vi "Prepare Loggers.vi"(6 "Groups":string[](array[string]), 8 "error in (no error)":errorcluster, 9 "Series":string, 10 "Folder":path, 11 "Log Manager Module in":refnum<class "Log Manager Module.lvclass">) -> (0 "error out":errorcluster, 3 "Log Manager Module out":refnum<class "Log Manager Module.lvclass">)   [LabVIEW 2020, in "VolatusData.lvlib" / "Log Manager Module.lvclass"]
uses:
  Log Manager Module.lvclass
  C:/dev/lv20CE/relink/lv-volatus/Volatus/Module/Module.lvclass
  Prepare Log.ctl
  Log Manager Module.lvclass/Log Manager Module.ctl
  Volatus/Event Level.ctl
  Volatus/Module/Module.lvclass/Module.ctl
  Logger State.ctl
  Volatus/Module/Module.lvclass
  VolatusData.lvlib
  Volatus/Volatus.lvlib
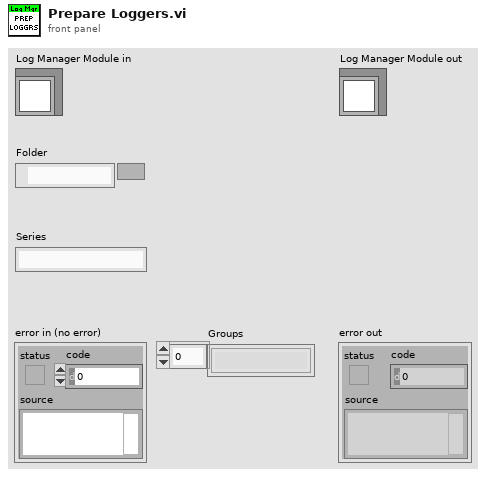
[diagram p1: front panel]
types:
  T1 = typedef "VolatusData.lvlib/Prepare Log.ctl" = cluster{"Folder":path, "Series":string}
  T2 = typedef "VolatusData.lvlib/Log Manager Module.lvclass/Group Info.ctl" = cluster{"Name":string, "Loggers":map{string, T3}}
  T3 = typedef "VolatusData.lvlib/Log Manager Module.lvclass/Logger.ctl" = cluster{"ID":string, "MsgQ":refnum<class "MessageQ.lvclass">, "State":T4, "Group":string}
  T4 = typedef "VolatusData.lvlib/Logger State.ctl" = enum16{"Unknown", "Idle", "Preparing", "Ready", "Logging", "Stopping"}
  T5 = typedef "Volatus.lvlib/Event Level.ctl" = enum16{"Debug", "Info", "Warning", "Error"}
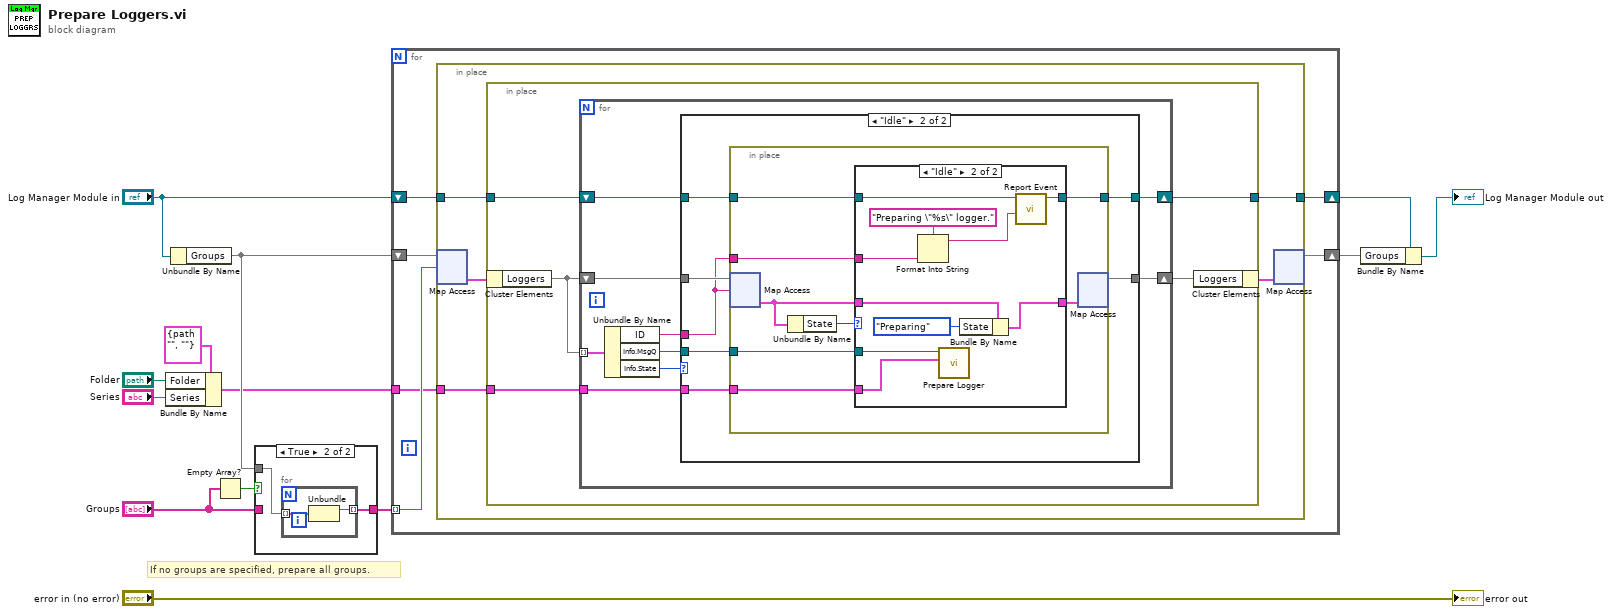
[diagram p0: block diagram]
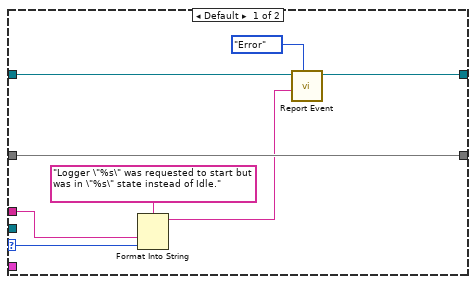
[diagram p2: hidden frame]
diagram:
  # "If no groups are specified, prepare all groups."
  n1 = Bundle By Name(cluster=T1 {"Folder"=path "", "Series"=""} ("Prepare Log"), "Folder"="Folder", "Series"="Series") -> (w1:T1)
  n2 = Unbundle By Name("Log Manager Module in") -> ("Groups"=w4:map{string, T2})
  n3 = Empty Array?(array="Groups") -> (empty?=w6:bool)
  n4 = case shown="True" w6 {
    tunnel: "Groups" -> [w14 _]
    tunnel: w4 -> [_ w16]
    tunnel: [w14 w15] -> w3
    frame False {
    }
    frame True {
      n5 = for {
        tunnel: w16 -> [w18] mode=indexing
        tunnel: [w17] -> w15 mode=indexing
        n6 = Unbundle(w18) -> ("Name"=w17:string)  [unwired: 1 out]
      }
    }
  }
  n7 = for {
    shift-right: [w23] -> w7
    shift-left: "Log Manager Module in" -> [w24]
    shift-right: [w20] -> w2
    shift-left: w4 -> [w22]
    tunnel: w3 -> [w21] mode=indexing
    tunnel: w1 -> [w19]
    n8 = in-place {
      in-place-border: w24 -> [w29]
      in-place-border: [w28] -> w23
      in-place-border: w19 -> [w25]
      n9 = in-place-map #1(w22, w21) -> (w27:T2)  [unwired: 1 in, 1 out]
      n10 = in-place {
        in-place-border: w29 -> [w34]
        in-place-border: [w33] -> w28
        in-place-border: w25 -> [w30]
        n11 = in-place-cluster #2(w27) -> ("Loggers"=w32:map{string, T3})
        n12 = for {
          tunnel: w32 -> [w43] mode=indexing
          shift-right: [w41] -> w31
          shift-left: w32 -> [w42]
          shift-right: [w38] -> w33
          shift-left: w34 -> [w39]
          tunnel: w30 -> [w35]
          n13 = Unbundle By Name(w43) -> ("ID"=w37:string, "Info.MsgQ"=w40:refnum<class "MessageQ.lvclass">, "Info.State"=w36:T4)
          n14 = case shown="\"Idle\"" w36 {
            selector: w36 -> [w46 _]
            tunnel: w42 -> [w49 w58]
            tunnel: [w49 w57] -> w41
            tunnel: w40 -> [_ w56]
            tunnel: w39 -> [w51 w55]
            tunnel: [w50 w54] -> w38
            tunnel: w37 -> [w45 w53]
            tunnel: w35 -> [_ w52]
            frame Default {
              n15 = Format Into String(format string="Logger \"%s\" was requested to start but was in \"%s\" state instead of Idle.", w45, w46) -> (resulting string=w44:string)  [unwired: 2 in, 1 out]
              n16 = call "Report Event.vi"("Level (Info)"=Event_Level."Error", "Message"=w44, "Module in"=w51) -> ("Module out"=w50:refnum<class "Log Manager Module.lvclass">)  [unwired: 7 in, 1 out]
            }
            frame "Idle" {
              n17 = in-place {
                in-place-border: w56 -> [w60]
                in-place-border: w55 -> [w64]
                in-place-border: [w63] -> w54
                in-place-border: w53 -> [w62]
                in-place-border: w52 -> [w59]
                n18 = in-place-map #3(w58, w53) -> (w65:T3)  [unwired: 1 in, 1 out]
                n19 = Unbundle By Name(w65) -> ("State"=w61:T4)
                n20 = case shown="\"Idle\"" w61 {
                  tunnel: [w67 w77] -> w66
                  tunnel: w65 -> [w67 w76]
                  tunnel: w64 -> [w68 w73]
                  tunnel: [w68 w72] -> w63
                  tunnel: w62 -> [_ w71]
                  tunnel: w60 -> [_ w70]
                  tunnel: w59 -> [_ w69]
                  frame Default {
                  }
                  frame "Idle" {
                    n21 = Format Into String(format string="Preparing \"%s\" logger.", w71) -> (resulting string=w75:string)  [unwired: 2 in, 1 out]
                    n22 = call "Prepare Logger.vi"("Prepare Log"=w69, "MsgQ in"=w70) -> ()  [unwired: 8 in, 2 out]
                    n23 = Bundle By Name(cluster=w76, "State"=Logger_State."Preparing") -> (w77:T3)
                    n24 = call "Report Event.vi"("Message"=w75, "Module in"=w73) -> ("Module out"=w72:refnum<class "Log Manager Module.lvclass">)  [unwired: 8 in, 1 out]
                  }
                }
                n25 = in-place-map #3(w66) -> (w57:map{string, T3})  [unwired: 1 in, 2 out]
              }
            }
          }
        }
        n26 = in-place-cluster #2("Loggers"=w31) -> (w26:T2)
      }
      n27 = in-place-map #1(w26) -> (w20:map{string, T2})  [unwired: 1 in, 2 out]
    }
  }
  n28 = Bundle By Name(cluster=w7, "Groups"=w2) -> (→"Log Manager Module out":refnum<class "Log Manager Module.lvclass">)
  "error out" <- "error in (no error)"
